vi "NT Read and Format Multiple Entries as String.vi"(8 "error in":errorcluster, 11 "Name Pattern":string) -> (0 "error out":errorcluster, 3 "Formatted Strings":cluster{"Name":string, "Value":string}[](array[cluster]))   [LabVIEW 2017]
doc: "Return the table entries that match the name pattern formatted into strings. Supported wildcards are * and ?."
uses:
  <vilib>/Rock Robotics/Network Tables/Make Table Operation.ctl
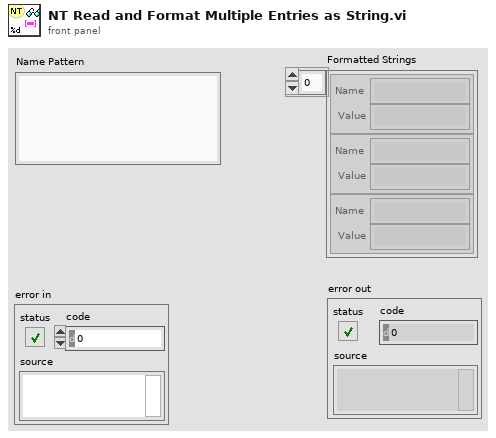
[diagram p1: front panel]
types:
  T1 = typedef "Make Table Operation.ctl" = enum16{"Get or Add Field", "Get Field or Add Temp", "Replace Temp ID", "Get Field ID - No Add", "Get Table Field IDs", "Get Field ID Info", "Move Field to Temp", "Validate", "Remove Field", "Remove All"}
  T2 = typedef "Field ID.ctl" = i32
  T3 = typedef "Field Data.ctl" = cluster{"Dbl":dbl, "String":string, "Type":T4, "Boolean":bool, "Sequence #":T5, "Flags":u8}
  T4 = typedef "Field Type.ctl" = enum8{"Invalid", "Bool", "Numeric", "String", "Raw", "Boolean Array", "Numeric Array", "String Array", "RPC"}
  T5 = typedef "Sequence.ctl" = u16
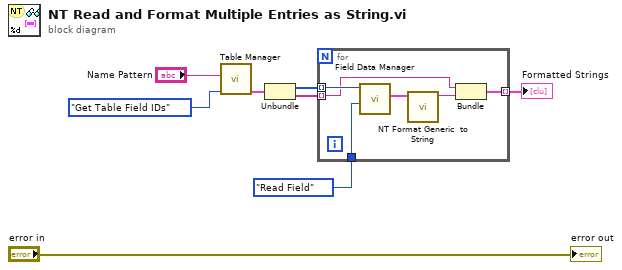
[diagram p0: block diagram]
diagram:
  n1 = call <vilib>:"Table Manager.vi"("Operation"=Make_Table_Operation."Get Table Field IDs", "Entry Name"="Name Pattern") -> ("Entries"=w4:cluster{"Entry IDs":T2[], "Names":string[]})  [unwired: 6 in, 3 out]
  n2 = Unbundle(w4) -> ("Entry IDs"=w3:T2[], "Names"=w1:string[])
  n3 = for {
    tunnel: w3 -> [w12] mode=indexing
    tunnel: [w10] -> w8 mode=indexing
    tunnel: enum16{"Update Field", "Read Field"}."Read Field" ("Operation") -> [w13]
    tunnel: w1 -> [w9] mode=indexing
    n4 = call <vilib>:"Field Data Manager.vi"("Operation"=w13, "Field ID"=w12) -> ("Field Value Out"=w14:T3)  [unwired: 8 in, 1 out]
    n5 = call <vilib>:"NT Format Generic  to String.vi"("Field Value"=w14) -> ("String"=w11:string)  [unwired: 10 in]
    n6 = Bundle("String"=w9, "String"=w11) -> (w10:cluster{"String":string, "String":string})  [unwired: 1 in]
  }
  "Formatted Strings" <- w8
  "error out" <- "error in"
